vi "Synchronize Caller Events.vi"(8 "error in":errorcluster, 11 "Module Admin":refnum<class "Delacor_lib_QMH_Cloneable Module Admin.lvclass">) -> (0 "error out":errorcluster, 3 "Module Admin out":refnum<class "Delacor_lib_QMH_Cloneable Module Admin.lvclass">)   [LabVIEW 2020, in "DAQ AI.lvlib"]
doc: "Synchronize with the caller of the module through the sequence of waiting on multiple rendezvous.\n_____\nBased on DQMH Dev Tools: Project Template 7.1.2.1547."
uses:
  DAQ AI.lvlib
  <vilib>/Delacor/Delacor QMH/Libraries/Cloneable Module Admin_class/Delacor_lib_QMH_Cloneable Module Admin.lvclass
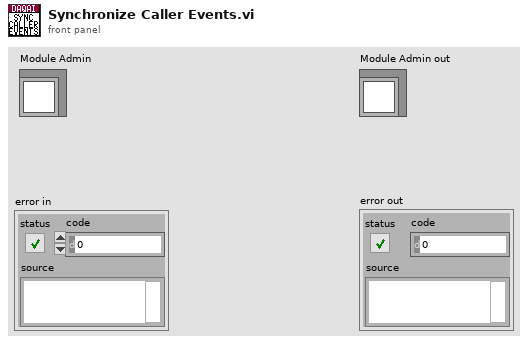
[diagram p1: front panel]
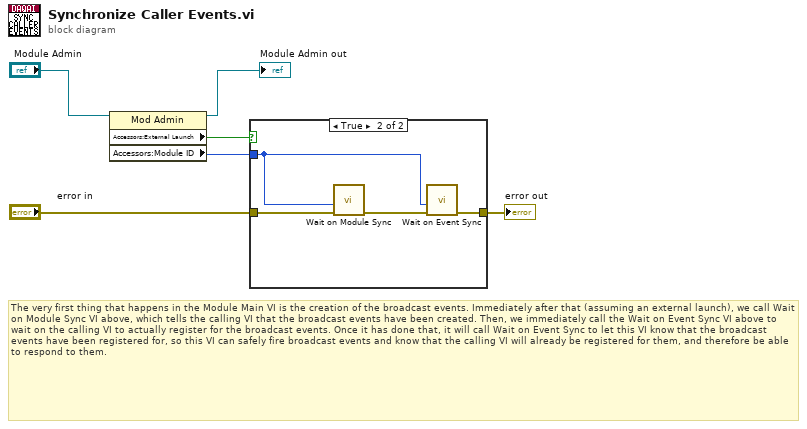
[diagram p0: block diagram]
diagram:
  # "The very first thing that happens in the Module Main VI is the creation of the broadcast events. Immediately after that (assuming an external launch), we call Wait on Module Sync VI above, which tells the calling VI that the broadcast events have been created. Then, we immediately call the Wait on Event Sync VI above to wait on the calling VI to actually register for the broadcast events. Once it has done that, it will call Wait on Event Sync to let this VI know that the broadcast events have been registered for, so this VI can safely fire broadcast events and know that the calling VI will already be registered for them, and therefore be able to respond to them."
  n1 = property class="Mod Admin"(reference="Module Admin") -> (reference out=→"Module Admin out":refnum<class "Delacor_lib_QMH_Cloneable Module Admin.lvclass">, "Accessors:External Launch"=w3:bool, "Accessors:Module ID"=w2:i32)  [unwired: 1 in, 1 out]
  n2 = case shown="True" w3 {
    tunnel: "error in" -> [w7 w11]
    tunnel: [w7 w9] -> w6
    tunnel: w2 -> [_ w8]
    frame False {
    }
    frame True {
      n3 = call "Wait on Module Sync.vi"("error in"=w11, "Module ID"=w8) -> ("error out"=w10:errorcluster)  [unwired: 9 in]
      n4 = call "Wait on Event Sync.vi"("error in"=w10, "Module ID"=w8) -> ("error out"=w9:errorcluster)  [unwired: 9 in]
    }
  }
  "error out" <- w6
